vi "toCluster.vi"(8 "error in (no error)":errorcluster, 11 "ACNET Device in":refnum<class "Copy of ACNET Device.lvclass">) -> (0 "error out":errorcluster, 2 "ACNET Device Cluster":T1, 3 "ACNET Device out":refnum<class "Copy of ACNET Device.lvclass">)   [LabVIEW 2013, in "Copy of ACNET Device.lvclass"]
uses:
  Copy of ACNET Device.lvclass
  Copy of ACNET Device.lvclass/Copy of ACNET Device.ctl
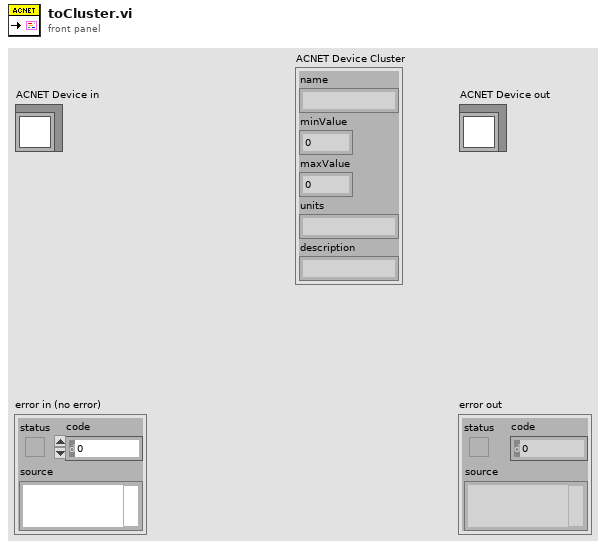
[diagram p1: front panel]
types:
  T1 = cluster{"name":string, "minValue":dbl, "maxValue":dbl, "units":string, "description":string}
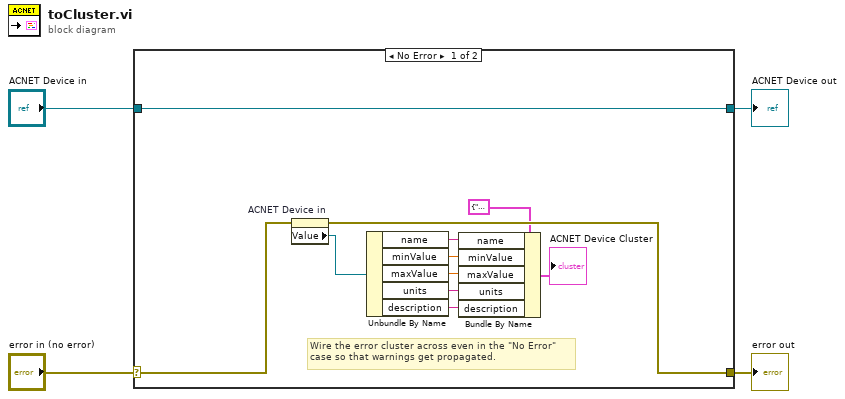
[diagram p0: block diagram]
diagram:
  n1 = case shown="No Error" "error in (no error)" {
    selector: "error in (no error)" -> [w14 w17]
    tunnel: [w13 w17] -> w3
    tunnel: [w15 w16] -> w1
    tunnel: "ACNET Device in" -> [w15 w16]
    frame No Error {
      # "Wire the error cluster across even in the \"No Error\"\ncase so that warnings get propagated."
      n2 = property on="ACNET Device in" class="LVClassControl (strict)"(error in=w14) -> (error out=w13:errorcluster, "Value"=w9:refnum<class "Copy of ACNET Device.lvclass">)  [unwired: 1 in, 1 out]
      n3 = Unbundle By Name(w9) -> ("name"=w12:string, "minValue"=w11:dbl, "maxValue"=w10:dbl, "units"=w8:string, "description"=w5:string)
      n4 = Bundle By Name(cluster=T1 {"name"="", "minValue"=0.0, "maxValue"=0.0, "units"="", "description"=""} ("ACNET Device Cluster"), "name"=w12, "minValue"=w11, "maxValue"=w10, "units"=w8, "description"=w5) -> (→"ACNET Device Cluster":T1)
    }
    frame Error {
    }
  }
  "error out" <- w3
  "ACNET Device out" <- w1
